vi "Research.vi"() -> ()   [LabVIEW 2014]
uses:
  <vilib>/httpClient/LabVIEWHTTPClient.lvlib
panel:
  out "body 2":string
  in  "Address":T1
  out "body":string
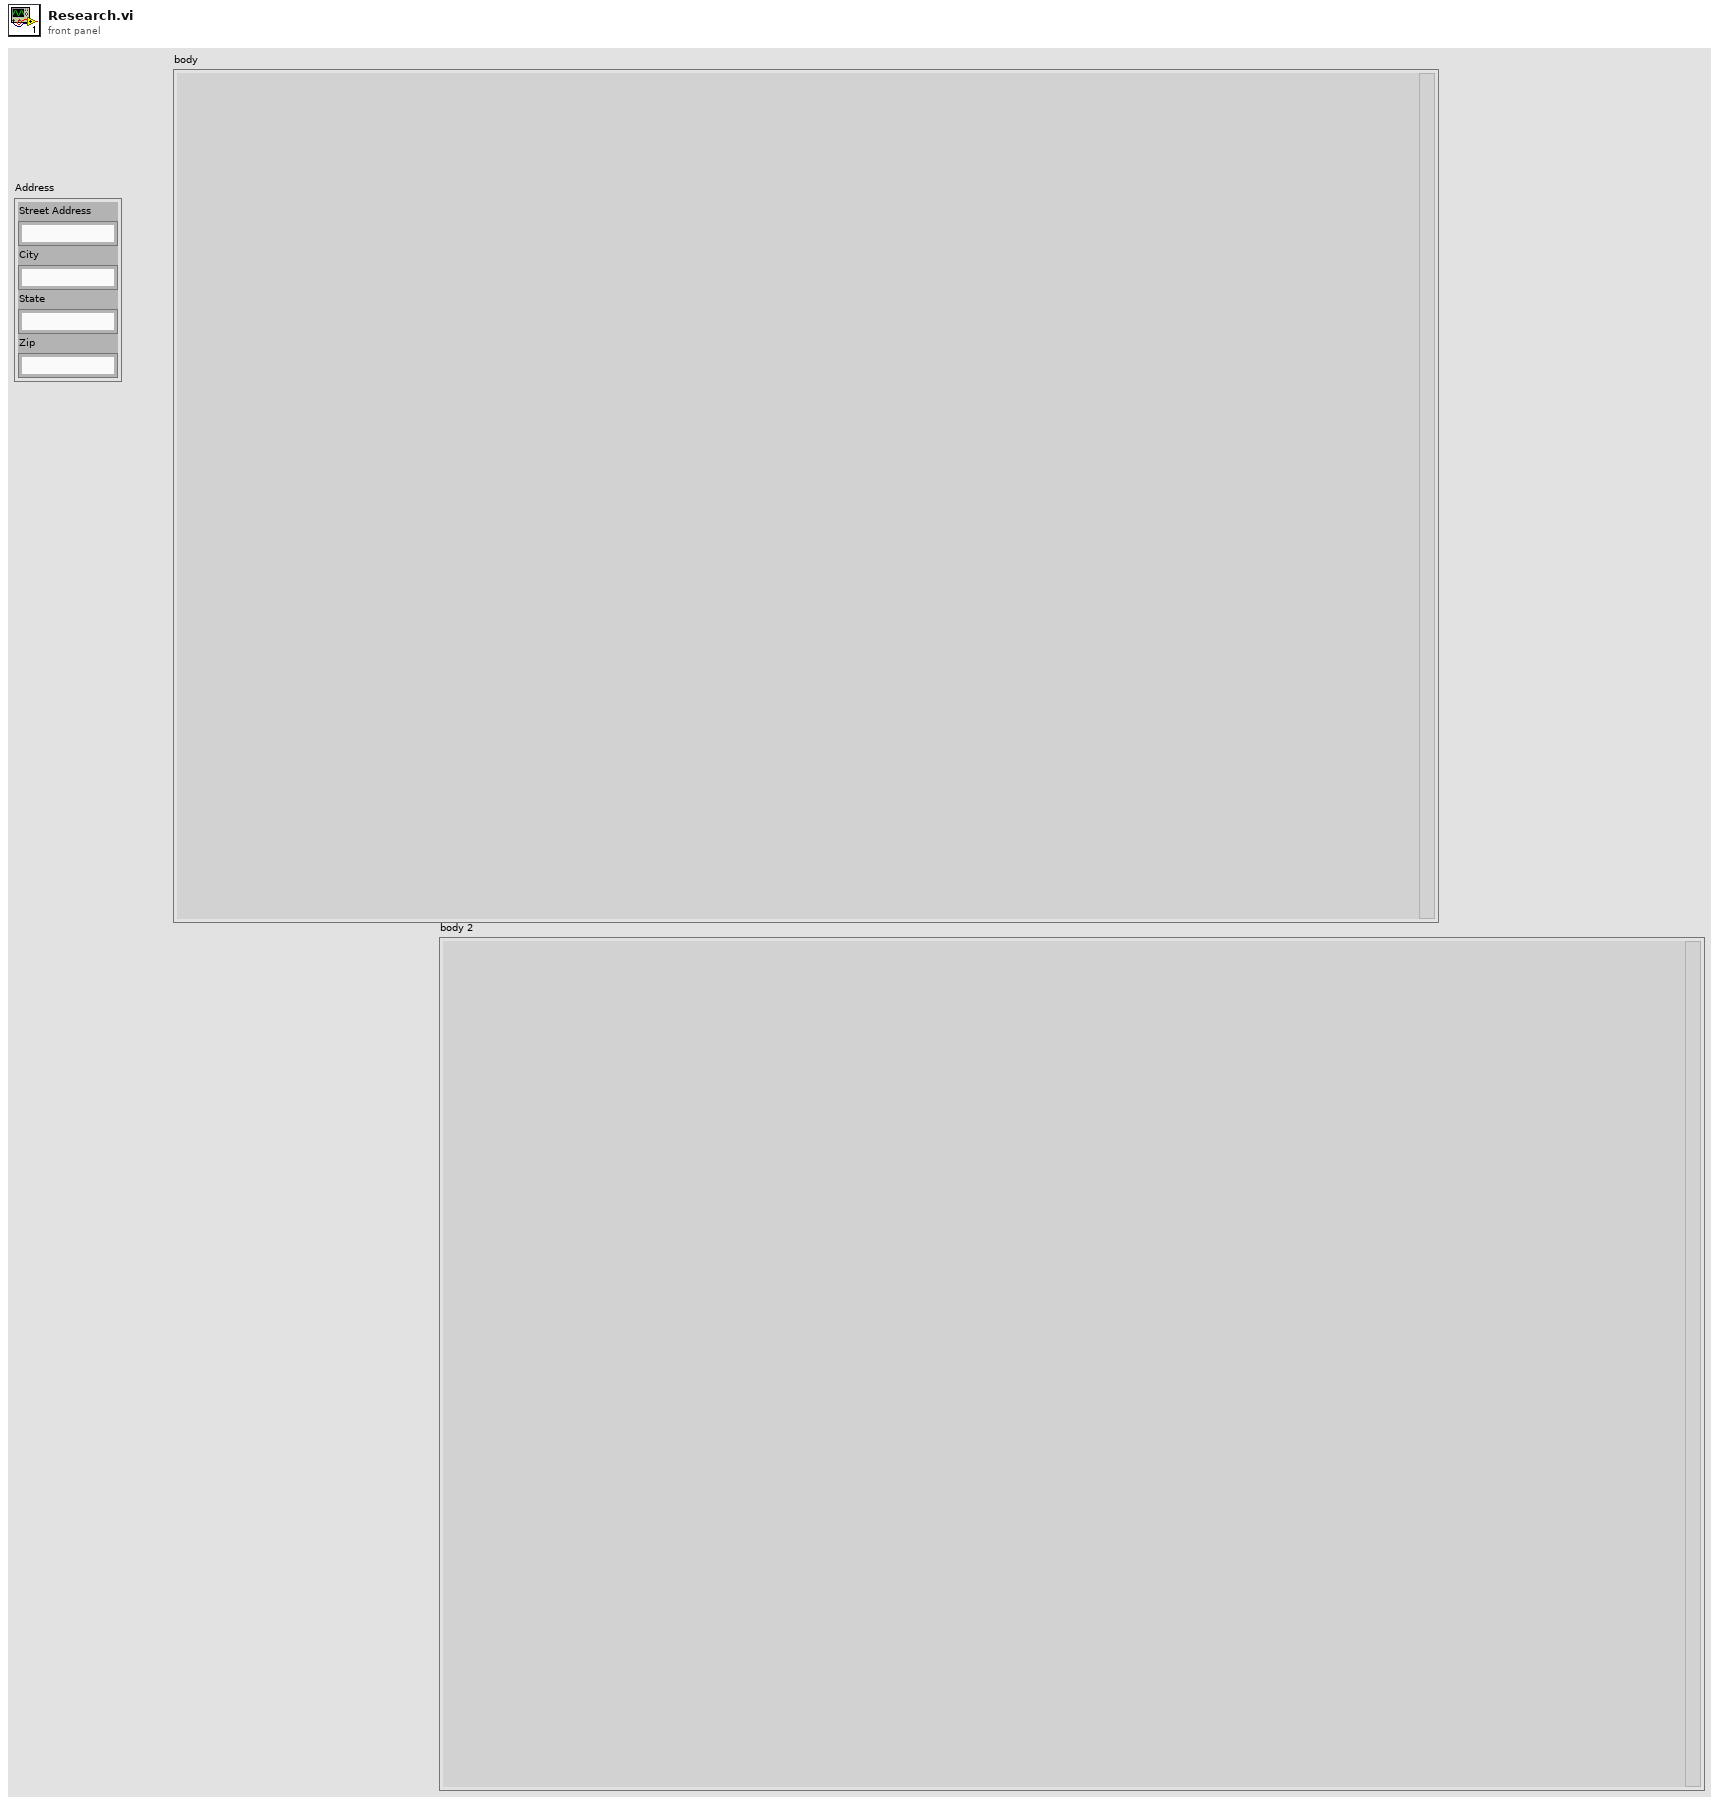
[diagram p1: front panel]
types:
  T1 = cluster{"Street Address":string, "City":string, "State":string, "Zip":string}
  T2 = typedef "LabVIEWHTTPClient.lvlib/ClientHandle.ctl" = refnum<k1>
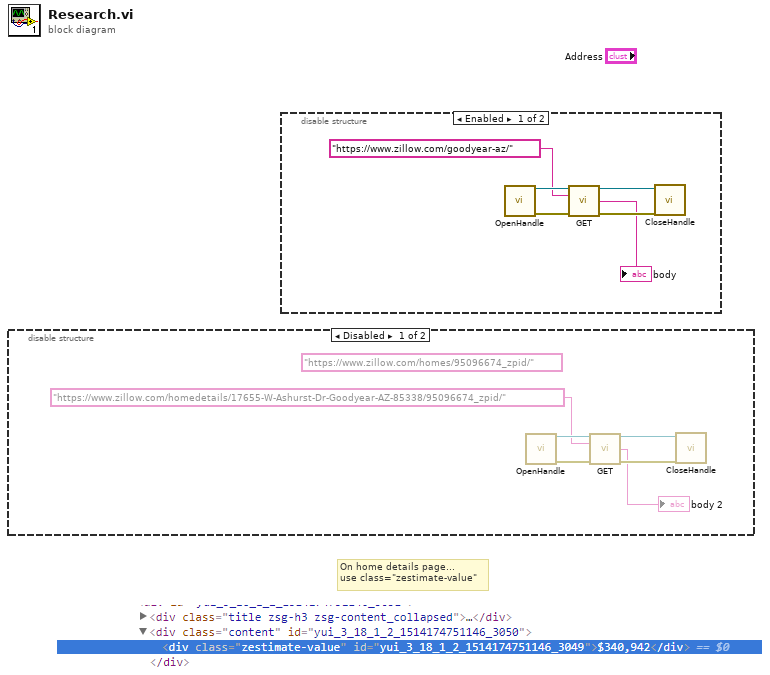
[diagram p0: block diagram]
diagram:
  # "On home details page...\nuse class=\"zestimate-value\""
  n1 = disable-structure shown="Disabled" {
    frame Disabled {
      (unwired) "https://www.zillow.com/homes/95096674_zpid/" ("url")
      n2 = call <vilib>:"OpenHandle.vi"() -> ("client handle out"=w3:T2, "error out"=w5:errorcluster)  [unwired: 14 in]
      n3 = call <vilib>:"GET.vi"("client handle"=w3, "url"="https://www.zillow.com/homedetails/17655-W-Ashurst-Dr-Goodyear-AZ-85338/95096674_zpid/", "error in (no error)"=w5) -> ("client handle out"=w6:T2, "body"=→"body 2":string, "error out"=w4:errorcluster)  [unwired: 9 in, 1 out]
      n4 = call <vilib>:"CloseHandle.vi"("client handle"=w6, "error in (no error)"=w4) -> ()  [unwired: 13 in, 1 out]
    }
    frame Enabled {
    }
  }
  n5 = disable-structure shown="Enabled" {
    frame Enabled {
      n6 = call <vilib>:"OpenHandle.vi"() -> ("client handle out"=w12:T2, "error out"=w9:errorcluster)  [unwired: 14 in]
      n7 = call <vilib>:"GET.vi"("client handle"=w12, "url"="https://www.zillow.com/goodyear-az/", "error in (no error)"=w9) -> ("client handle out"=w7:T2, "body"=→"body":string, "error out"=w10:errorcluster)  [unwired: 9 in, 1 out]
      n8 = call <vilib>:"CloseHandle.vi"("client handle"=w7, "error in (no error)"=w10) -> ()  [unwired: 13 in, 1 out]
    }
    frame Disabled {
    }
  }
